vi "DB posting example.vi"(8 "error in":errorcluster, 11 "Data cluster to be posted":T1) -> (0 "error IO":errorcluster)   [LabVIEW 2012]
uses:
  Nick's small accelerator db/nick typedef.ctl
  <vilib>/addons/database/NI_Database_API.lvlib
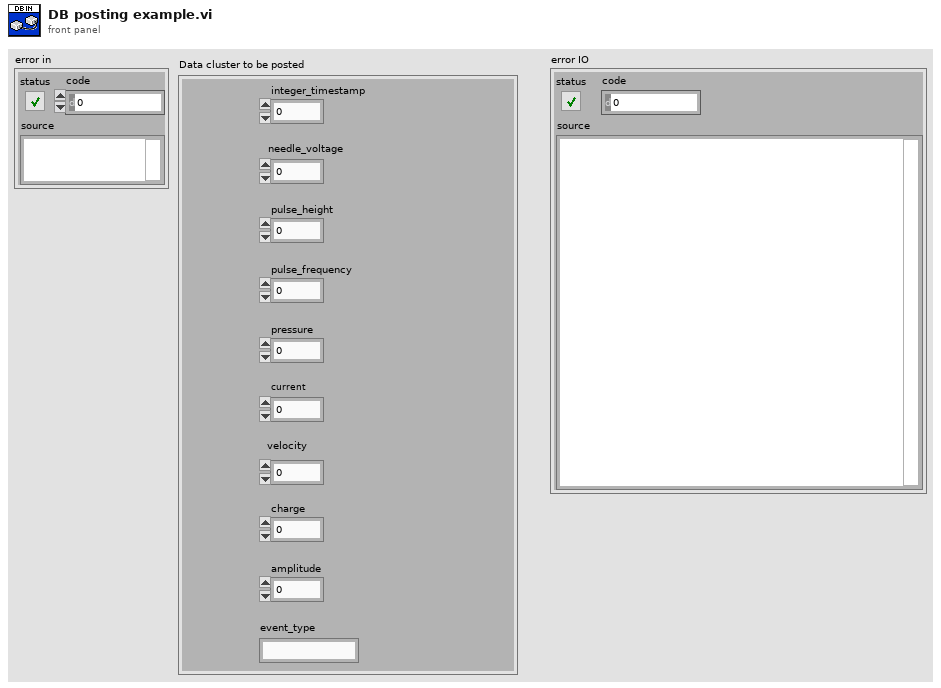
[diagram p1: front panel]
types:
  T1 = typedef "nick typedef.ctl" = cluster{"integer_timestamp":i64, "needle_voltage":dbl, "pulse_height":dbl, "pulse_frequency":dbl, "pressure":dbl, "current":dbl, "velocity":dbl, "charge":dbl, "amplitude":dbl, "event_type":string}
  T2 = typedef "NI_Database_API.lvlib/Conn ObjectReference.ctl" = refnum<k1>
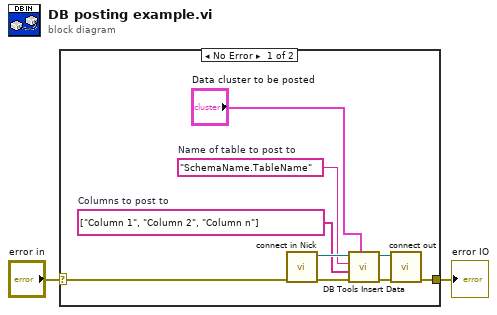
[diagram p0: block diagram]
diagram:
  n1 = case shown="No Error" "error in" {
    selector: "error in" -> [w10 w12]
    tunnel: [w11 w12] -> w1
    frame No Error {
      w3 = string[] ["Column 1", "Column 2", "Column n"]  # Columns to post to
      w6 = "SchemaName.TableName"  # Name of table to post to
      n2 = call "connect in Nick.vi"("error in (no error)"=w10) -> ("error out"=w8:errorcluster, "Database Connection"=w9:T2)  [unwired: 7 in]
      n3 = call <vilib>:"DB Tools Insert Data.vi"("data"="Data cluster to be posted", "error in (no error)"=w8, "columns"=w3, "table"=w6, "connection reference"=w9) -> ("error out"=w4:errorcluster, "connection reference out"=w7:T2)  [unwired: 5 in]
      n4 = call "connect out.vi"("error in (no error)"=w4, "connection reference"=w7) -> ("error out"=w11:errorcluster)  [unwired: 9 in]
    }
    frame Error {
    }
  }
  "error IO" <- w1
